vi "WF0_Hout_Lout.vi"(5 "Num_Read":i32) -> (0 "D-mode":string[](array[string]), 2 "B-mode":string[](array[string]))   [LabVIEW 2016]
uses:
  TemperatureMeasure/Thermal_type.vi
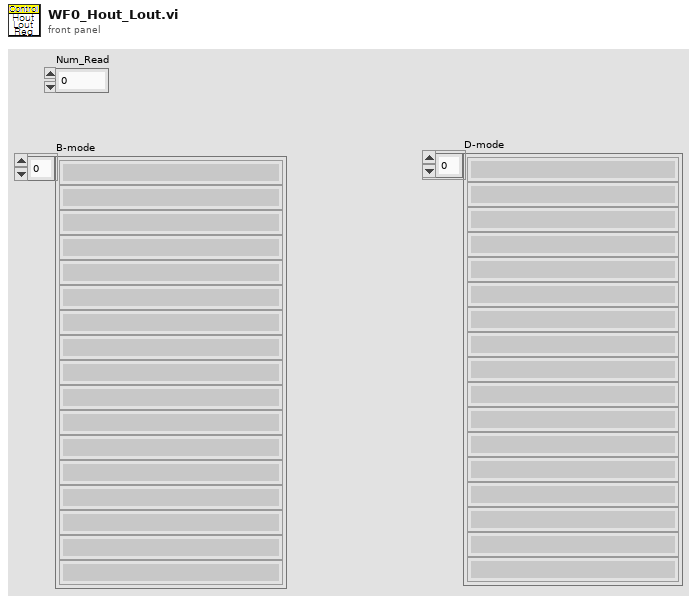
[diagram p1: front panel]
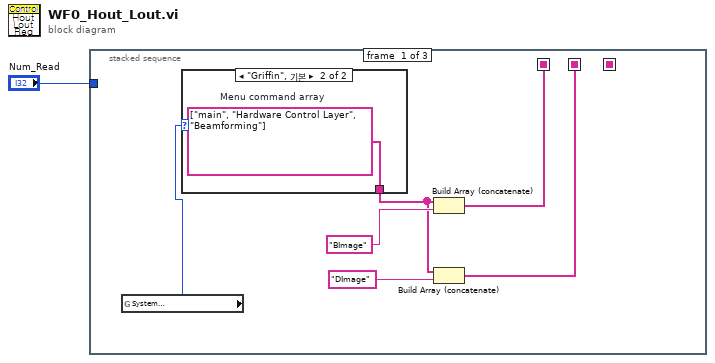
[diagram p0: block diagram]
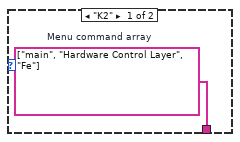
[diagram p2: hidden frame]
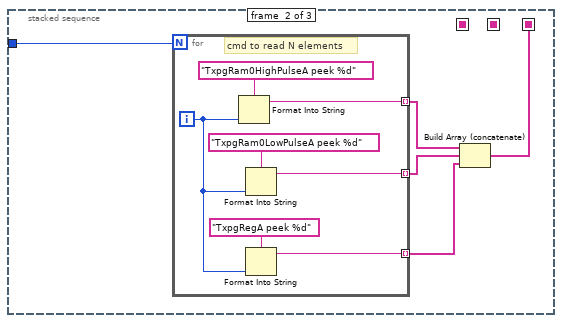
[diagram p3: hidden frame]
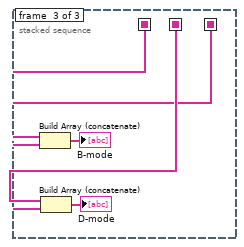
[diagram p4: hidden frame]
diagram:
  n1 = stacked-sequence {
    seq-local: [w4 _ _] -> [_ _ w26]
    seq-local: [w3 _ _] -> [_ _ w25]
    seq-local: [_ w11 _] -> [_ _ w24]
    tunnel: "Num_Read" -> [_ w10 _]
    frame #0 {
      n2 = global read "Thermal_type.vi" "System \nSelection"() -> (w2:enum32{"Common", "Frosk", "Griffin", "K2"})
      n3 = case shown="\"Griffin\", 기본" w2 {
        tunnel: [w8 w9] -> w6
        frame "K2" {
          w8 = string[] ["main", "Hardware Control Layer", "Fe"]  # Menu command array
        }
        frame "Griffin", Default {
          w9 = string[] ["main", "Hardware Control Layer", "Beamforming"]  # Menu command array
        }
      }
      n4 = Build Array (concatenate)(w6, "BImage") -> (w4:string[])
      n5 = Build Array (concatenate)(w6, "DImage") -> (w3:string[])
    }
    frame #1 {
      n6 = for {
        N: w10 -> [_]
        tunnel: [w17] -> w14 mode=indexing
        tunnel: [w16] -> w13 mode=indexing
        tunnel: [w15] -> w12 mode=indexing
        i -> [w18]
        # "cmd to read N elements"
        n7 = Format Into String(format string="TxpgRam0HighPulseA peek %d" ("Format String"), w18) -> (resulting string=w17:string)  [unwired: 2 in, 1 out]
        n8 = Format Into String(format string="TxpgRam0LowPulseA peek %d" ("Format String"), w18) -> (resulting string=w16:string)  [unwired: 2 in, 1 out]
        n9 = Format Into String(format string="TxpgRegA peek %d" ("Format String"), w18) -> (resulting string=w15:string)  [unwired: 2 in, 1 out]
      }
      n10 = Build Array (concatenate)(w14, w13, w12) -> (w11:string[])
    }
    frame #2 {
      n11 = Build Array (concatenate)(w26, w24) -> (→"B-mode":string[])
      n12 = Build Array (concatenate)(w25, w24) -> (→"D-mode":string[])
    }
  }
